vi "GetGObjects_FP_DigitalDisplays.vi"(8 "error in":errorcluster, 11 "VI Interpreter in":refnum<class "VI Interpreter.lvclass">) -> (0 "error out":errorcluster, 3 "VI Interpreter out":refnum<class "VI Interpreter.lvclass">)   [LabVIEW 2014, in "Raspberry Pi Compatible Compiler for LabVIEW.lvlib" / "VI Interpreter.lvclass"]
uses:
  VI Interpreter.lvclass
  <vilib>/Utility/traverseref.llb/TRef TravTarget.ctl
  VI Interpreter.lvclass/VI Interpreter.ctl
  GObject/GObject.lvclass
  <vilib>/Utility/traverseref.llb/VI Scripting - Traverse.lvlib
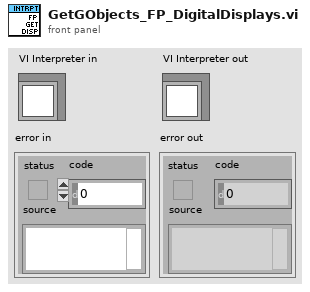
[diagram p1: front panel]
types:
  T1 = typedef "TRef TravTarget.ctl" = enum16{"FP", "BD", "Other"}
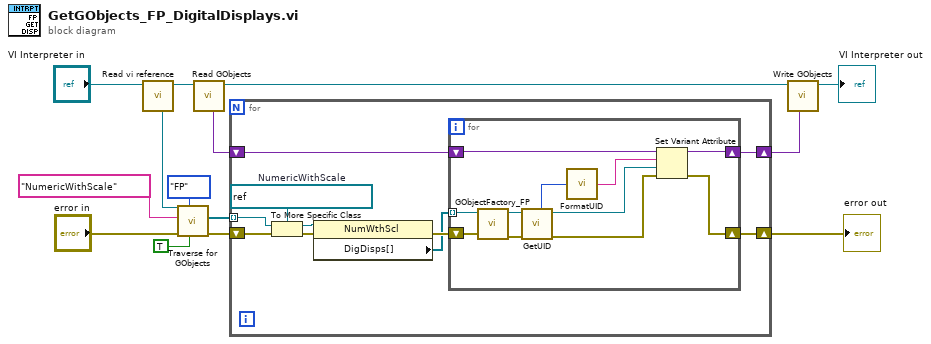
[diagram p0: block diagram]
diagram:
  n1 = call "Read vi reference.vi"("VI Interpreter in"="VI Interpreter in") -> ("VI Interpreter out"=w3:refnum<class "VI Interpreter.lvclass">, "vi reference"=w9:refnum<vi>)  [unwired: 7 in]
  n2 = call <vilib>:"Traverse for GObjects.vi"("Traverse Generated Code (F)"=TRUE, "Traverse Target"=TRef_TravTarget."FP", "error in (no error)"="error in", "Class Name"="NumericWithScale", "VI Refnum"=w9) -> ("error out"=w13:errorcluster, "References"=w12:refnum<vi>[])  [unwired: 3 in, 2 out]
  n3 = call "Read GObjects.vi"("VI Interpreter in"=w3) -> ("VI Interpreter out"=w2:refnum<class "VI Interpreter.lvclass">, "GObjects"=w1:variant)  [unwired: 7 in]
  n4 = for {
    tunnel: w12 -> [w20] mode=indexing
    shift-right: [w23] -> w7
    shift-left: w13 -> [w21]
    shift-right: [w22] -> w6
    shift-left: w1 -> [w24]
    w19 = refnum<vi> refnum  # NumericWithScale
    n5 = To More Specific Class(target class=w19, reference=w20, error in=w21) -> (specific class reference=w18:refnum<vi>, error out=w17:errorcluster)
    n6 = property class="NumWthScl"(reference=w18, error in=w17) -> (error out=w16:errorcluster, "DigDisps[]"=w15:refnum<vi>[])  [unwired: 1 out]
    n7 = for {
      tunnel: w15 -> [w25] mode=indexing
      shift-right: [w35] -> w22
      shift-left: w24 -> [w34]
      shift-right: [w33] -> w23
      shift-left: w16 -> [w31]
      n8 = call "GObjectFactory_FP.vi"("error in"=w31, "reference"=w25) -> ("error out"=w30:errorcluster, "GObject out"=w29:refnum<class "GObject.lvclass">)  [unwired: 8 in]
      n9 = call-dynamic "GetUID.vi"("error in"=w30, "GObject in"=w29) -> ("error out"=w26:errorcluster, "GObject out"=w27:refnum<class "GObject.lvclass">, "UID"=w28:i32)  [unwired: 5 in]
      n10 = call "FormatUID.vi"("UID"=w28) -> ("Name"=w32:string)
      n11 = Set Variant Attribute(Variant=w34, name=w32, value=w27, error in=w26) -> (Variant out=w35:variant, error out=w33:errorcluster)  [unwired: 1 out]
    }
  }
  "error out" <- w7
  n12 = call "Write GObjects.vi"("GObjects"=w6, "VI Interpreter in"=w2) -> ("VI Interpreter out"=→"VI Interpreter out":refnum<class "VI Interpreter.lvclass">)  [unwired: 7 in]
